vi "checkFinishDirectEnemyPlay.vi"(8 "error in (no error)":errorcluster, 9 "last command_interpreted":T1, 10 "Game":refnum<class "Game.lvclass">, 11 "DirectEnemyPlay in":refnum<class "DirectEnemyPlay.lvclass">) -> (0 "error out":errorcluster, 2 "Boolean":bool, 3 "DirectEnemyPlay out":refnum<class "DirectEnemyPlay.lvclass">)   [LabVIEW 2018, in "DirectEnemyPlay.lvclass"]
uses:
  DirectEnemyPlay.lvclass
  Game_class/Game.lvclass
  Referee_class/command_interpreted.ctl
  Game_class/Game.lvclass/Game.ctl
  Referee_class/Referee.lvclass/Referee.ctl
  Events_class/Events.lvclass/Events.ctl
  Game_class/Read Referee.vi
  Game_class/Read EventsRef.vi
  Game_class/Read EnemyRef.vi
  Events_class/Read ball_out.vi
  Events_class/Read kick.vi
  Referee_class/Read command_interpreted.vi
  Referee_class/Referee.lvclass
  Events_class/Events.lvclass
  Enemy_class/Enemy.lvclass
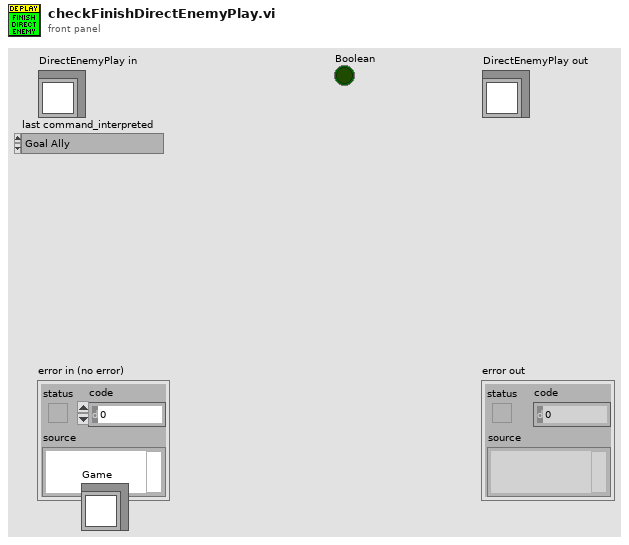
[diagram p1: front panel]
types:
  T1 = typedef "command_interpreted.ctl" = enum16{"Goal Ally", "Goal Enemy", "Ball Placement Enemy", "Ball Placement Ally", "Normal Half Time", "Extra Time  Break", "Extra Half Time", "None", "Post Game", "PKA Normal Start", "Prepare Kickoff Ally", "PKE Normal Start", "Prepare Kickoff Enemy", "Force Start", "Halt", "Timeout", "Prepare Penalty Ally", "Prepare Penalty Enemy", "PPA NormalStart", "PPE Normal Start", "Indirect Free Ally", "Direct Free Enemy", "Direct Free Ally", "Indirect Free Enemy", "Stop"}
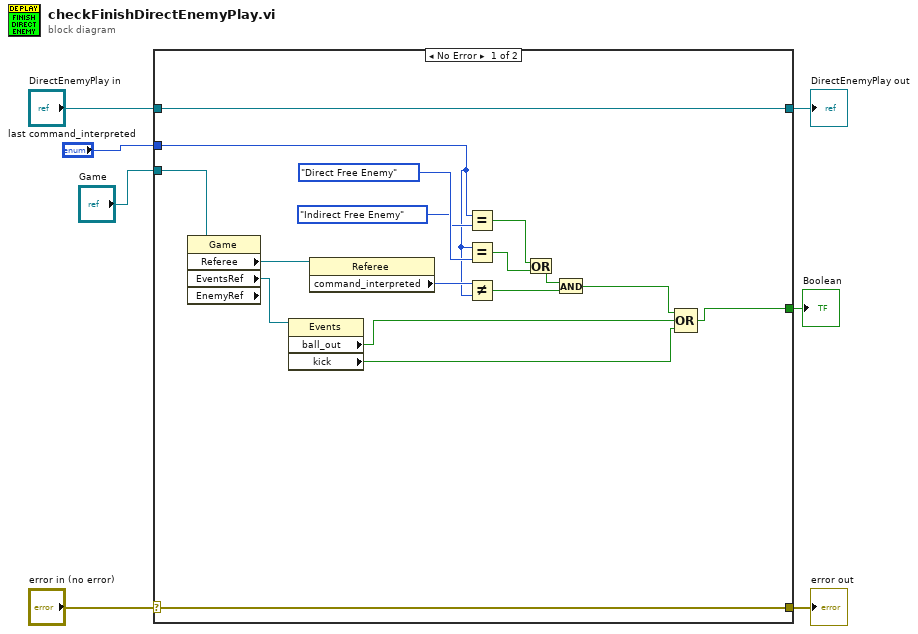
[diagram p0: block diagram]
diagram:
  n1 = case shown="No Error" "error in (no error)" {
    selector: "error in (no error)" -> [w23 w26]
    tunnel: [w23 w26] -> w6
    tunnel: [w24 w25] -> w4
    tunnel: "DirectEnemyPlay in" -> [w24 w25]
    tunnel: "Game" -> [w18 _]
    tunnel: [w14 _] -> w2
    tunnel: "last command_interpreted" -> [w8 _]
    frame No Error {
      n2 = property class="Game" props=["Referee", "EventsRef", "EnemyRef"](reference=w18) -> ("Referee"=w22:refnum<class "Referee.lvclass">, "EventsRef"=w17:refnum<class "Events.lvclass">)  [unwired: 1 in, 3 out]
      n3 = property class="Events"(reference=w17) -> ("ball_out"=w15:bool, "kick"=w13:bool)  [unwired: 1 in, 2 out]
      n4 = property class="Referee"(reference=w22) -> ("command_interpreted"=w20:T1)  [unwired: 1 in, 2 out]
      n5 = Equal?(x=w8, y=command_interpreted."Indirect Free Enemy" ("command_interpreted")) -> (x = y?=w10:bool)
      n6 = Equal?(x=w8, y=command_interpreted."Direct Free Enemy" ("command_interpreted")) -> (x = y?=w11:bool)
      n7 = Not Equal?(x=w20, y=w8) -> (x != y?=w19:bool)
      n8 = Or(x=w10, y=w11) -> (x .or. y?=w12:bool)
      n9 = And(x=w12, y=w19) -> (x .and. y?=w16:bool)
      n10 = Compound Arithmetic op=OR(w16, w15, w13) -> (w14:bool)
    }
    frame Error {
    }
  }
  "error out" <- w6
  "DirectEnemyPlay out" <- w4
  "Boolean" <- w2
